vi "Load Top-Level VI.vi"() -> ()   [LabVIEW 2023]
panel:
  out "error out":errorcluster
  # "Loading User Interface, Please Wait..."
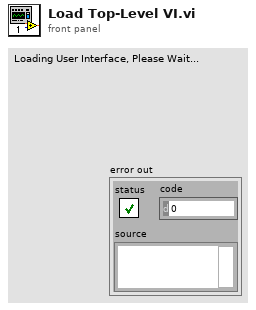
[diagram p1: front panel]
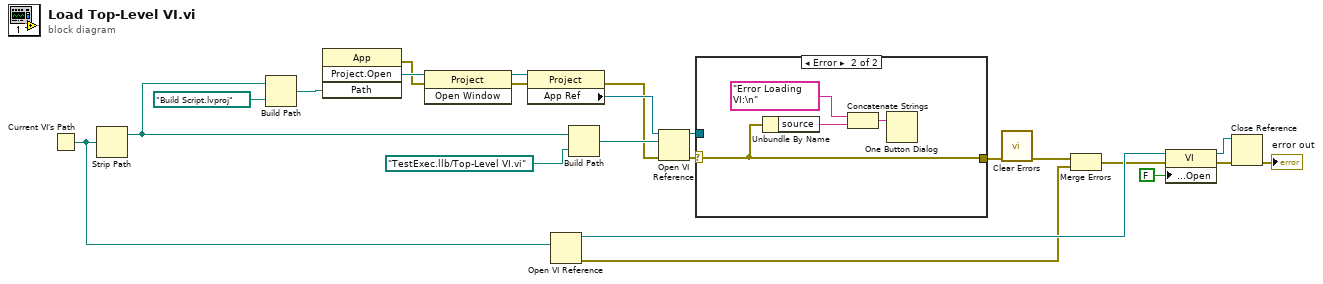
[diagram p0: block diagram]
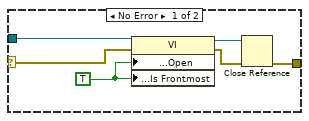
[diagram p2: hidden frame]
diagram:
  n1 = Current VI's Path() -> (path=w14:path)
  n2 = Strip Path(path=w14) -> (stripped path=w12:path)  [unwired: 1 out]
  n3 = Build Path(base path=w12, name or relative path=path "Build Script.lvproj") -> (appended path=w11:path)
  n4 = invoke class="App" method="Project.Open"("Path"=w11) -> (error out=w4:errorcluster, "Project:Open"=w6:refnum<vi>)  [unwired: 3 in, 2 out]
  n5 = invoke class="Project" method="Open Window"(reference=w6, error in=w4) -> (reference out=w5:refnum<vi>, error out=w3:errorcluster)  [unwired: 1 in, 1 out]
  n6 = property class="Project"(reference=w5, error in=w3) -> (error out=w10:errorcluster, "App Ref"=w13:refnum<vi>)  [unwired: 1 out]
  n7 = Open VI Reference(vi path=w14) -> (vi reference=w18:refnum<vi>, error out=w8:errorcluster)  [unwired: 1 in, 4 out]
  n8 = Build Path(base path=w12, name or relative path=path "TestExec.llb/Top-Level VI.vi") -> (appended path=w23:path)
  n9 = Open VI Reference(application reference (local)=w13, vi path=w23, error in (no error)=w10) -> (vi reference=w22:refnum<vi>, error out=w21:errorcluster)  [unwired: 3 out]
  n10 = case shown="Error" w21 {
    selector: w21 -> [w25 w30]
    tunnel: w22 -> [w29 _]
    tunnel: [w24 w30] -> w20
    frame No Error {
      w28 = TRUE ("Front Panel Window:Open")
      n11 = property class="VI"(reference=w29, error in=w25, "Front Panel Window:Open"=w28, "Front Panel Window:Is Frontmost"=w28) -> (reference out=w27:refnum<vi>, error out=w26:errorcluster)
      n12 = Close Reference(reference=w27, error in (no error)=w26) -> (error out=w24:errorcluster)
    }
    frame Error {
      n13 = Unbundle By Name(w30) -> ("source"=w33:string)
      n14 = Concatenate Strings("Error Loading VI:\n" ("string"), w33) -> (w31:string)
      n15 = One Button Dialog(message=w31) -> ()  [unwired: 2 out]
    }
  }
  n16 = call <vilib>:"Clear Errors.vi"("error in (no error)"=w20) -> ("error out"=w9:errorcluster)  [unwired: 1 in, 5 out]
  n17 = Merge Errors(w9, w8) -> (w7:errorcluster)
  n18 = property class="VI"(reference=w18, error in=w7, "Front Panel Window:Open"=FALSE) -> (reference out=w16:refnum<vi>, error out=w17:errorcluster)
  n19 = Close Reference(reference=w16, error in (no error)=w17) -> (error out=→"error out":errorcluster)
